vi "LS370Monitor_test.vi"(6 "still automatic":bool=TRUE, 8 "wait for T":bool=TRUE, 9 "Heater Off":bool=TRUE, 10 "Rate K/min":dbl, 11 "Setpoint LS370":dbl) -> (2 "Heater \nPower (W)":dbl, 3 "MC Temperature":dbl=291.191)   [LabVIEW 2016]
uses:
  Instrument_Setup_v2.vi
  data/Data_Display_global.vi
panel:
  out "MC Resistance":dbl=291.191
  out "FilmBurner heater (W)":dbl=1.0 format="%^_3e"
  in  "FilmBurner (mA)":dbl=1.0
  out "Nr. of cycles":i32
  in  "MC Thermometer":u16(ring)=2 items=["Speer S9905"=1, "Rox U02453"=2]
  out "Still heater (W)":dbl=1.0 format="%^_3e"
  in  "LS370 \nAuto Excitation":bool
  in  "Update every [ms]":dbl=1000.0 min=0.0 max=60000.0 step=500.0
  out "Auto\nExcitation":bool
  in  "Update every [ms] 2":dbl=60000.0 min=0.0 max=60000.0 step=500.0
  in  "Still value (mA)":dbl=3.0
  in  "T(K) still=on?":dbl=0.7
  out "?":bool
  out "?":bool
  out "?":bool
  in  "sweep\ntolerance %":dbl=0.1
  in  "stability \ntolerance (%)":dbl=0.5
  out "stability (K)":dbl
  out "Aktuelle Zeit":timestamp[](array[timestamp])
  out "Excitation AVS":dbl
  out "Excitation LS":dbl
  out "MC Temp kleiner als":dbl
  in  "stop":bool
  out "Temperature":cluster{timestamp[], dbl[]}[](graph)
  out "Heater Power":cluster{timestamp[], dbl[]}(graph)
  out "Offset new SP":dbl
  out "Heater Range":dbl
  out "P (Gain)":dbl
  out "I (Reset)":dbl
  out "D (Rate)":dbl
  out "HeaterTableLS370.txt":string caption="PID Table"
  out "Pfad zu HeaterTable":path=path "C:/01_Mischer_control/CryoTUM_Mischer_Version_2-0/HeaterTableLS370-highT"
  # "PID Control"
  # "Normal \noperation"
  # "Still control"
  # "0: Off\n1: 10mW\n2: 100mW\n3: 1.0W\n4: 10W"
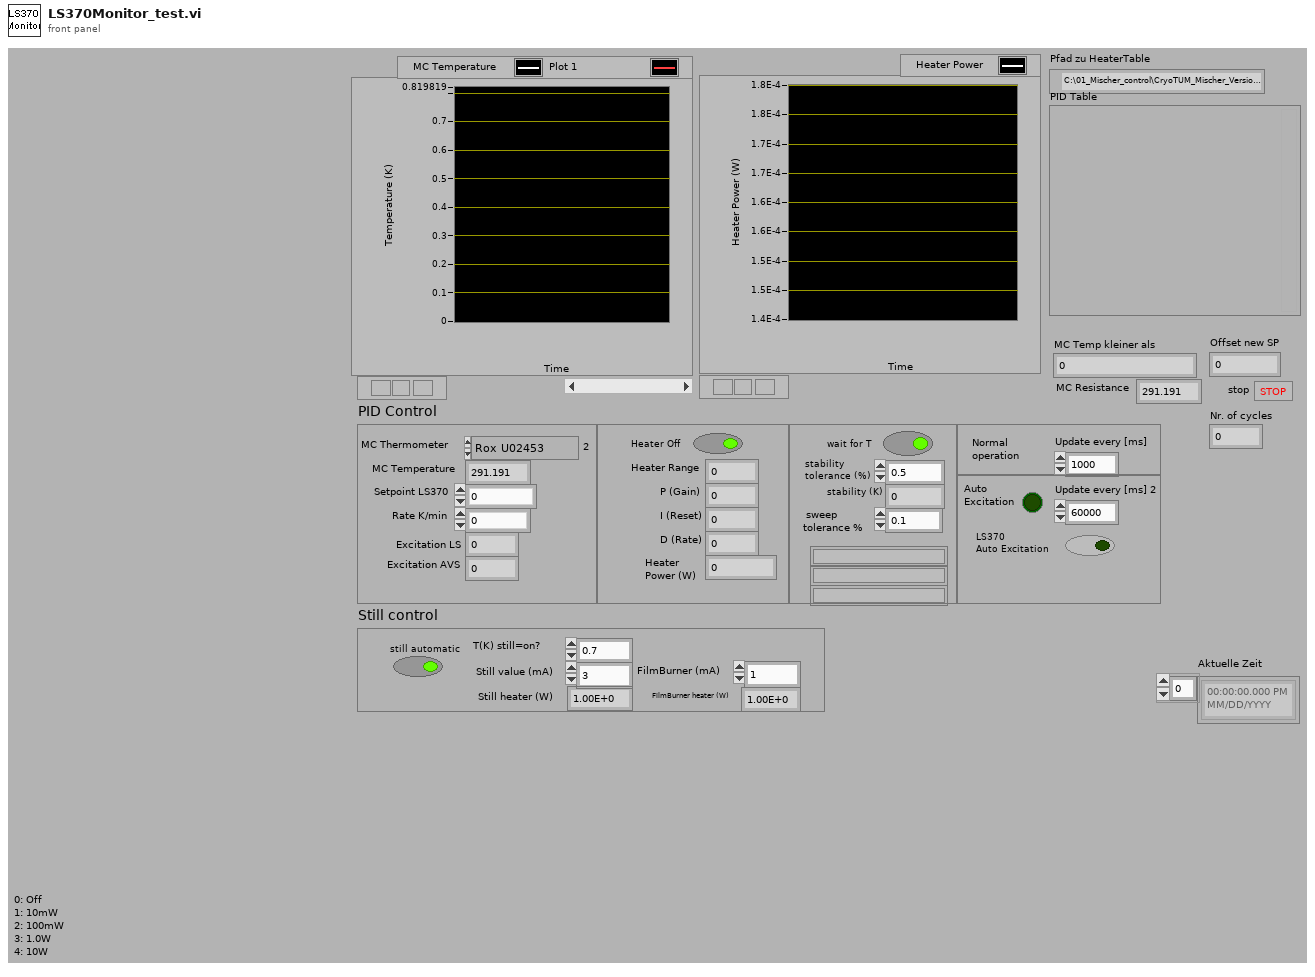
[diagram p1: front panel]
types:
  T1 = enum16{"open", "replace", "create", "open or create", "replace or create", "replace or create with confirmation"}
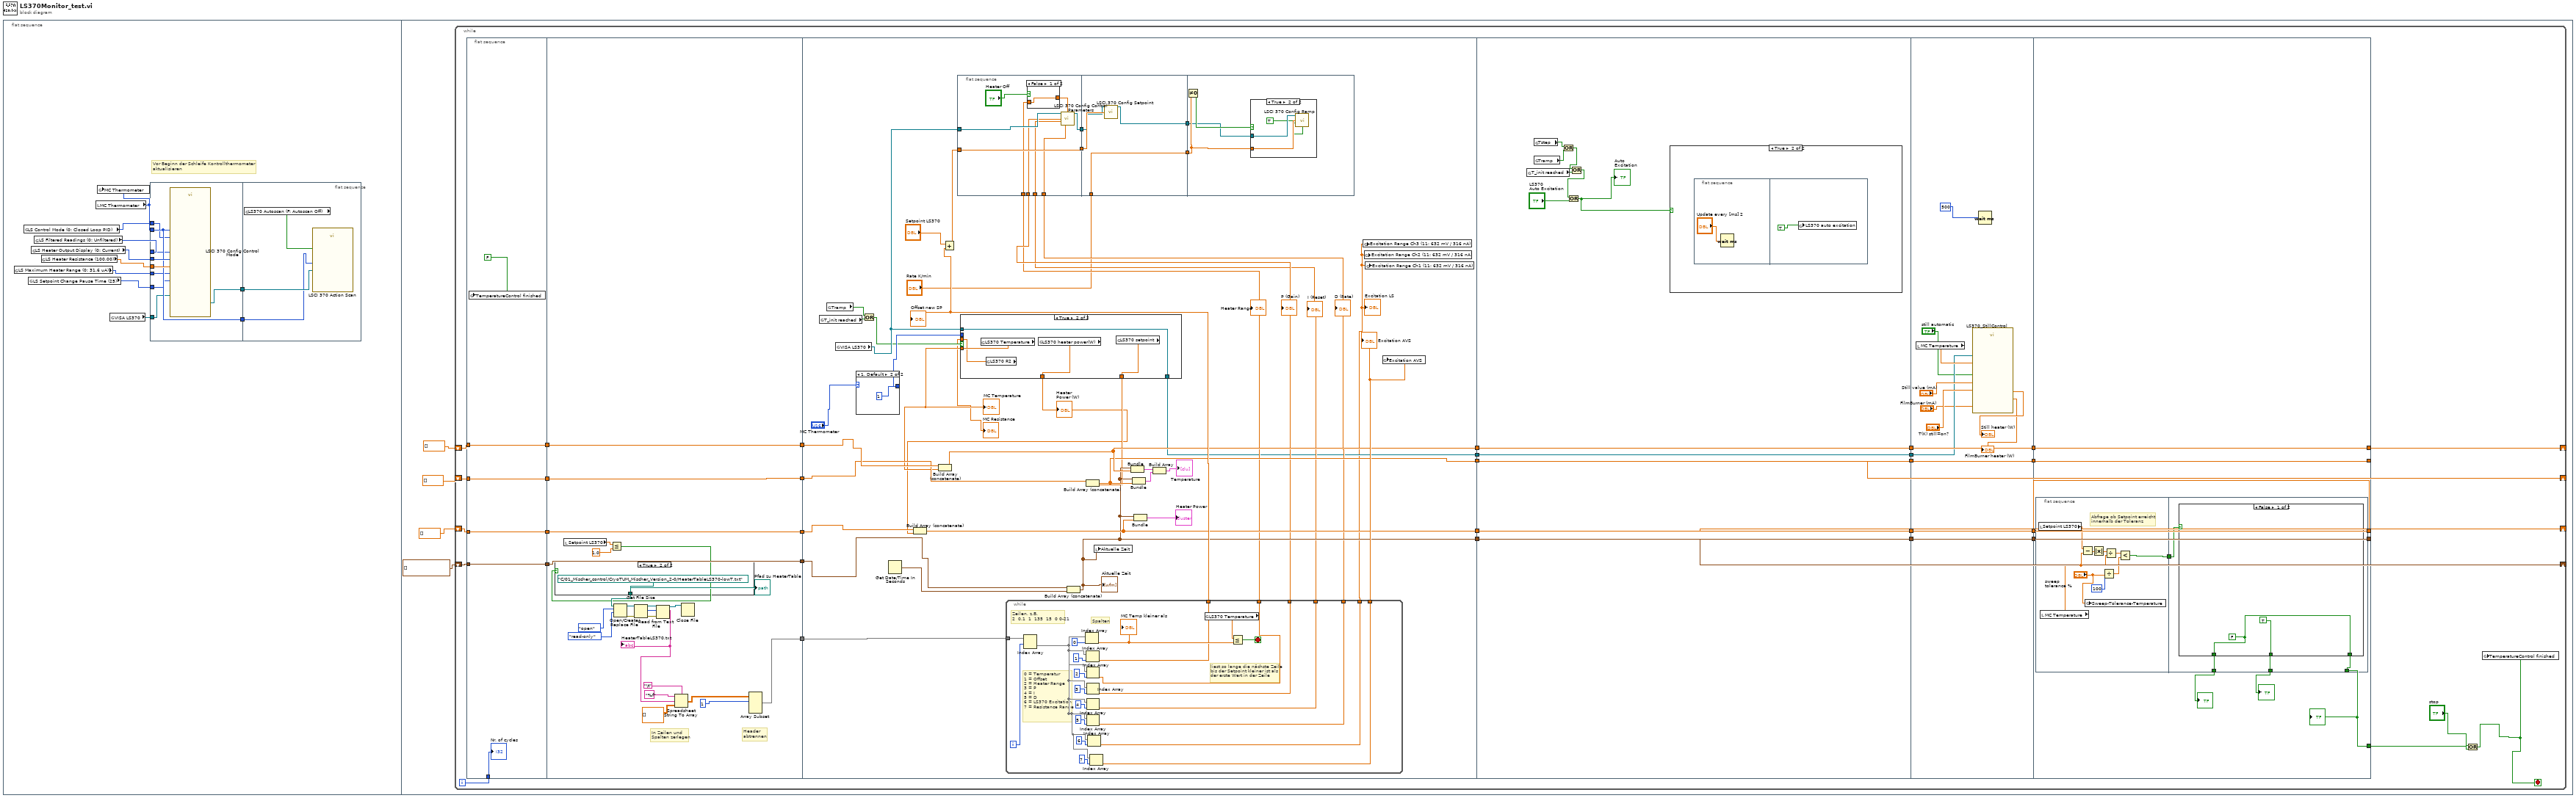
[diagram p0: block diagram]
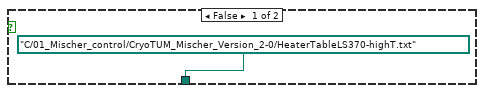
[diagram p2: hidden frame]
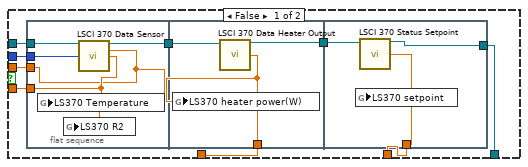
[diagram p3: hidden frame]
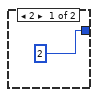
[diagram p4: hidden frame]
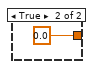
[diagram p5: hidden frame]
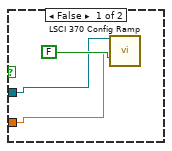
[diagram p6: hidden frame]
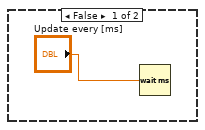
[diagram p7: hidden frame]
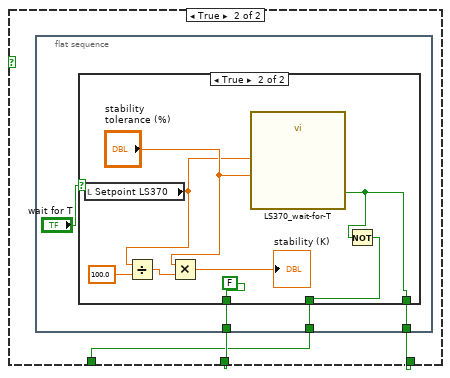
[diagram p8: hidden frame]
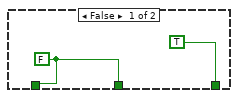
[diagram p9: hidden frame]
diagram:
  n1 = flat-sequence {
    frame #0 {
      # "Vor Beginn der Schleife Kontrollthermometer \naktualisieren"
      n2 = global read "Instrument_Setup_v2.vi" "LS Maximum Heater Range (0: 31.6 uA)"() -> (w2:u16)
      n3 = global read "Instrument_Setup_v2.vi" "LS Control Mode (0: Closed Loop PID)"() -> (w1:u16)
      n4 = global read "Instrument_Setup_v2.vi" "LS Setpoint Change Pause Time (25)"() -> (w3:i32)
      n5 = global read "Instrument_Setup_v2.vi" "LS Heater Output Display (0: Current)"() -> (w5:u16)
      n6 = global read "Instrument_Setup_v2.vi" "LS Filtered Readings (0: Unfiltered)"() -> (w6:u16)
      n7 = global read "Instrument_Setup_v2.vi" "LS Heater Resistance (100.00)"() -> (w4:dbl)
      n8 = local read "MC Thermometer"() -> (w7:u16)
      n9 = global write "Instrument_Setup_v2.vi" "MC Thermometer"(w7) -> ()
      n10 = global read "Instrument_Setup_v2.vi" "VISA LS370"() -> (w10:refnum<visa-resource-name>)
      n11 = flat-sequence {
        tunnel: w10 -> [w13]
        tunnel: w7 -> [w17]
        tunnel: w4 -> [w19]
        tunnel: w5 -> [w18]
        tunnel: [w17] -> w9
        tunnel: [w16] -> w8
        tunnel: w6 -> [w15]
        tunnel: w3 -> [w14]
        tunnel: w2 -> [w12]
        tunnel: w1 -> [w11]
        tunnel: w9 -> [w21]
        tunnel: w8 -> [w22]
        frame #0 {
          n12 = call "LSCI 370 Config Control Mode.vi"("VISA session"=w13, "Setpoint Change\nPause Time (25)"=w14, "Control Mode (0: Closed Loop PID)"=w11, "Channel (1)"=w17, "Filtered Readings (0: Unfiltered)"=w15, "Heater Output Display (0: Current)"=w18, "Heater Resistance (100.00)"=w19, "Maximum Heater Range (0: 31.6 uA)"=w12) -> ("dup VISA session"=w16:refnum<visa-resource-name>)  [unwired: 6 in, 1 out]
        }
        frame #1 {
          n13 = global read "Instrument_Setup_v2.vi" "LS370 Autoscan (F: Autoscan Off)"() -> (w20:bool)
          n14 = call "LSCI 370 Action Scan.vi"("VISA session"=w22, "Scan Channel (1)"=w21, "Autoscan (F: Autoscan Off)"=w20) -> ()  [unwired: 11 in, 2 out]
        }
      }
    }
    frame #1 {
      n15 = while {
        shift-right: [w54] -> _
        shift-left: dbl[] [] -> [w50]
        shift-right: [w53] -> _
        shift-left: timestamp[] [] -> [w49]
        shift-right: [w55] -> _
        shift-left: dbl[] [] -> [w51]
        shift-right: [w56] -> _
        shift-left: dbl[] [] -> [w52]
        i -> [w31]
        stop <- w29 stop-if-true
        n16 = flat-sequence {
          tunnel: w49 -> [w64]
          tunnel: w50 -> [w65]
          tunnel: w51 -> [w66]
          tunnel: w52 -> [w67]
          tunnel: [w67] -> w48
          tunnel: [w66] -> w47
          tunnel: [w65] -> w46
          tunnel: [w64] -> w45
          tunnel: w31 -> [w62]
          tunnel: [w76] -> w61
          tunnel: [w75] -> w60
          tunnel: [w74] -> w59
          tunnel: [w73] -> w58
          tunnel: [w72] -> w57
          tunnel: w48 -> [w75]
          tunnel: w47 -> [w74]
          tunnel: w46 -> [w73]
          tunnel: w45 -> [w72]
          tunnel: w61 -> [w131]
          tunnel: w60 -> [w122]
          tunnel: w59 -> [w121]
          tunnel: w58 -> [w120]
          tunnel: w57 -> [w119]
          tunnel: [w118] -> w40
          tunnel: [w117] -> w38
          tunnel: [w116] -> w36
          tunnel: [w115] -> w34
          tunnel: [w100] -> w32
          tunnel: w40 -> [w215]
          tunnel: [w215] -> w39
          tunnel: w38 -> [w214]
          tunnel: [w214] -> w37
          tunnel: w36 -> [w213]
          tunnel: [w213] -> w35
          tunnel: w34 -> [w212]
          tunnel: [w212] -> w33
          tunnel: w32 -> [w207]
          tunnel: [w207] -> w27
          tunnel: w39 -> [w231]
          tunnel: [w231] -> w44
          tunnel: w37 -> [w230]
          tunnel: [w230] -> w43
          tunnel: w35 -> [w229]
          tunnel: [w229] -> w42
          tunnel: w33 -> [w228]
          tunnel: [w228] -> w41
          tunnel: w27 -> [w224]
          tunnel: [w236] -> w53
          tunnel: [w237] -> w54
          tunnel: [w238] -> w55
          tunnel: [w239] -> w56
          tunnel: w44 -> [w239]
          tunnel: w43 -> [w238]
          tunnel: w42 -> [w237]
          tunnel: w41 -> [w236]
          tunnel: [w232] -> _
          tunnel: [w232] -> w30
          frame #0 {
            n17 = global write "Instrument_Setup_v2.vi" "TemperatureControl finished"(FALSE) -> ()
            "Nr. of cycles" <- w62
          }
          frame #1 {
            # "In Zeilen und \nSpalten zerlegen"
            # "Header\nabtrennen"
            n18 = local read "Setpoint LS370"() -> (w70:dbl)
            n19 = Less Or Equal?(x=w70, y=1.0) -> (x <= y?=w68:bool)
            n20 = case shown="True" w68 {
              tunnel: [path "C:/01_Mischer_control/CryoTUM_Mischer_Version_2-0/HeaterTableLS370-highT.txt" path "C:/01_Mischer_control/CryoTUM_Mischer_Version_2-0/HeaterTableLS370-lowT.txt"] -> w71
              frame False {
              }
              frame True {
              }
            }
            "Pfad zu HeaterTable" <- w71
            n21 = Open/Create/Replace File(file path (use dialog)=w71, operation (0:open)=T1."open", access (0:read/write)=enum16{"read/write", "read-only", "write-only"}."read-only") -> (refnum out=w86:refnum<file>, error out=w88:errorcluster)  [unwired: 3 in, 1 out]
            n22 = Get File Size(file=w86, error in=w88) -> (refnum out=w85:refnum<file>, size (in bytes)=w81:i64, 0:w87:errorcluster)
            n23 = Read from Text File(file (use dialog)=w85, count=w81, error in=w87) -> (refnum out=w84:refnum<file>, text=w80:string)  [unwired: 1 in, 2 out]
            "HeaterTableLS370.txt" <- w80
            n24 = Spreadsheet String To Array(delimiter (Tab)="\t", format string="%f", spreadsheet string=w80, array type (2D Dbl)=dbl[][] []) -> (array=w79:dbl[][])
            n25 = Close File(refnum=w84) -> ()  [unwired: 1 in, 2 out]
            n26 = Array Subset(array=w79, index (row)=1) -> (w76:dbl[][])  [unwired: 3 in]
          }
          frame #2 {
            n27 = global read "Data_Display_global.vi" "T_init reached"() -> (w97:bool)
            n28 = global read "Data_Display_global.vi" "Tramp"() -> (w96:bool)
            n29 = global read "Instrument_Setup_v2.vi" "VISA LS370"() -> (w102:refnum<visa-resource-name>)
            n30 = case shown="1, Default" "MC Thermometer" {
              tunnel: [2 1] -> w103
              frame 2 {
              }
              frame 1, Default {
              }
            }
            n31 = Or(x=w96, y=w97) -> (x .or. y?=w95:bool)
            n32 = Get Date/Time In Seconds() -> (seconds since 1Jan1904=w126:timestamp)
            n33 = flat-sequence {
              tunnel: [w167] -> w108
              tunnel: w113 -> [w165]
              tunnel: w112 -> [w164]
              tunnel: w111 -> [w163]
              tunnel: w110 -> [w162]
              tunnel: [w160] -> w107
              tunnel: w128 -> [w167]
              tunnel: w102 -> [w166]
              tunnel: w108 -> [w173]
              tunnel: [w170] -> w109
              tunnel: w107 -> [w172]
              tunnel: [w171] -> w106
              tunnel: "Rate K/min" -> [w170]
              tunnel: w109 -> [w175]
              tunnel: w106 -> [w174]
              frame #0 {
                n34 = case shown="False" "Heater Off" {
                  tunnel: w162 -> [w168 _]
                  tunnel: [w168 0.0] -> w161
                  frame False {
                  }
                  frame True {
                  }
                }
                n35 = call "LSCI 370 Config Control Parameters.vi"("VISA session"=w166, "Heater Range (0: Off)"=w161, "Gain (P) (10.000)"=w165, "Reset (I) (20)"=w164, "Rate (D) (0)"=w163) -> ("dup VISA session"=w160:refnum<visa-resource-name>)  [unwired: 9 in, 1 out]
              }
              frame #1 {
                n36 = call "LSCI 370 Config Setpoint.vi"("VISA session"=w172, "Setpoint (0.00000E+0)"=w173) -> ("dup VISA session"=w171:refnum<visa-resource-name>)  [unwired: 12 in, 1 out]
              }
              frame #2 {
                n37 = Not Equal To 0?(x=w175) -> (x != 0?=w176:bool)
                n38 = case shown="True" w176 {
                  tunnel: w174 -> [w178 w182]
                  tunnel: w175 -> [w177 w181]
                  frame False {
                    n39 = call "LSCI 370 Config Ramp.vi"("VISA session"=w178, "Rate Value (0.001)"=w177, "Ramping On/Off (F: Ramping Off)"=FALSE) -> ()  [unwired: 11 in, 2 out]
                  }
                  frame True {
                    n40 = call "LSCI 370 Config Ramp.vi"("VISA session"=w182, "Rate Value (0.001)"=w181, "Ramping On/Off (F: Ramping Off)"=TRUE) -> ()  [unwired: 11 in, 2 out]
                  }
                }
              }
            }
            n41 = case shown="True" w95 {
              tunnel: w103 -> [w138 _]
              tunnel: w102 -> [w137 w153]
              tunnel: [w136 w154] -> w101
              tunnel: [w135 w153] -> w100
              tunnel: [w134 w156] -> w99
              tunnel: [w133 w155] -> w98
              tunnel: [w132 w152] -> w94
              frame False {
                n42 = flat-sequence {
                  tunnel: w138 -> [w145]
                  tunnel: w137 -> [w144]
                  tunnel: [w143] -> w140
                  tunnel: [w142] -> w134
                  tunnel: [w141] -> w132
                  tunnel: w140 -> [w148]
                  tunnel: [w146] -> w133
                  tunnel: [w147] -> w139
                  tunnel: [w149] -> w136
                  tunnel: w139 -> [w151]
                  tunnel: [w150] -> w135
                  frame #0 {
                    n43 = call "LSCI 370 Data Sensor.vi"("VISA session"=w144, "Channel (1)"=w145) -> ("dup VISA session"=w143:refnum<visa-resource-name>, "Resistance Reading"=w141:dbl, "Kelvin Reading"=w142:dbl)  [unwired: 9 in, 2 out]
                    n44 = global write "Data_Display_global.vi" "LS370 Temperature"(w142) -> ()
                    n45 = global write "Data_Display_global.vi" "LS370 R2"(w141) -> ()
                  }
                  frame #1 {
                    n46 = call "LSCI 370 Data Heater Output.vi"("VISA session"=w148) -> ("dup VISA session"=w147:refnum<visa-resource-name>, "Heater Output"=w146:dbl)  [unwired: 12 in, 1 out]
                    n47 = global write "Data_Display_global.vi" "LS370 heater power(W)"(w146) -> ()
                  }
                  frame #2 {
                    n48 = call "LSCI 370 Status Setpoint.vi"("VISA session"=w151) -> ("dup VISA session"=w150:refnum<visa-resource-name>, "Setpoint (0.00000E+0)"=w149:dbl)  [unwired: 12 in, 1 out]
                    n49 = global write "Data_Display_global.vi" "LS370 setpoint"(w149) -> ()
                  }
                }
              }
              frame True {
                n50 = global read "Data_Display_global.vi" "LS370 Temperature"() -> (w156:dbl)
                n51 = global read "Data_Display_global.vi" "LS370 R2"() -> (w152:dbl)
                n52 = global read "Data_Display_global.vi" "LS370 heater power(W)"() -> (w155:dbl)
                n53 = global read "Data_Display_global.vi" "LS370 setpoint"() -> (w154:dbl)
              }
            }
            "MC Temperature" <- w99
            "Heater \nPower (W)" <- w98
            "MC Resistance" <- w94
            n54 = Build Array (concatenate)(w120, w98) -> (w116:dbl[])
            n55 = Build Array (concatenate)(w122, w99) -> (w118:dbl[])
            n56 = while {
              tunnel: w131 -> [w203]
              tunnel: [w194] -> w129
              tunnel: [w192] -> w110
              tunnel: [w191] -> w113
              tunnel: [w190] -> w112
              tunnel: [w189] -> w111
              tunnel: [w187] -> w93
              tunnel: [w184] -> w127
              i -> [w202]
              stop <- w196 stop-if-true
              # "0 = Temperatur\n1 = Offset\n2 = Heater Range\n3 = P\n4 = I\n5 = D\n6 = LS370 Excitation\n7 = Resistance Range"
              # "liest so lange die nächste Zeile\nbis der Setpoint kleiner ist als \nder erste Wert in der Zeile"
              # "Zeilen, z.B. \n2  0.1  1  135  15  0 0-21"
              # "Spalten"
              n57 = Index Array(array=w203, index (row)=w202) -> (element=w185:dbl[])  [unwired: 1 in]
              n58 = Index Array(array=w185, index=0) -> (element=w195:dbl)
              "MC Temp kleiner als" <- w195
              n59 = Index Array(array=w185, index=1) -> (element=w194:dbl)
              n60 = Index Array(array=w185, index=2) -> (element=w192:dbl)
              n61 = Index Array(array=w185, index=3) -> (element=w191:dbl)
              n62 = Index Array(array=w185, index=4) -> (element=w190:dbl)
              n63 = Index Array(array=w185, index=5) -> (element=w189:dbl)
              n64 = Index Array(array=w185, index=6) -> (element=w187:dbl)
              n65 = Index Array(array=w185, index=7) -> (element=w184:dbl)
              n66 = global read "Data_Display_global.vi" "LS370 Temperature"() -> (w183:dbl)
              n67 = Less Or Equal?(x=w183, y=w195) -> (x <= y?=w196:bool)
            }
            "Offset new SP" <- w129
            "Heater Range" <- w110
            "P (Gain)" <- w113
            "I (Reset)" <- w112
            "D (Rate)" <- w111
            "Excitation LS" <- w93
            "Excitation AVS" <- w127
            n68 = Add(x="Setpoint LS370", y=w129) -> (x+y=w128:dbl)
            n69 = Build Array (concatenate)(w119, w126) -> (w115:timestamp[])
            "Aktuelle Zeit" <- w115
            n70 = Build Array (concatenate)(w121, w101) -> (w117:dbl[])
            n71 = local write "Aktuelle Zeit"(w115) -> ()
            n72 = Bundle(w115, w118) -> (w125:cluster{timestamp[], dbl[]})  [unwired: 1 in]
            n73 = Bundle(w115, w117) -> (w123:cluster{timestamp[], dbl[]})  [unwired: 1 in]
            n74 = Bundle(w115, w116) -> (→"Heater Power":cluster{timestamp[], dbl[]})  [unwired: 1 in]
            n75 = Build Array(w125, w123) -> (→"Temperature":cluster{timestamp[], dbl[]}[])
            n76 = global write "Instrument_Setup_v2.vi" "Excitation Range Ch3 (11: 632 mV / 316 nA)"(w93) -> ()
            n77 = global write "Instrument_Setup_v2.vi" "Excitation Range Ch2 (11: 632 mV / 316 nA)"(w93) -> ()
            n78 = global write "Instrument_Setup_v2.vi" "Excitation Range Ch1 (11: 632 mV / 316 nA)"(w93) -> ()
            n79 = global write "Instrument_Setup_v2.vi" "Excitation AVS"(w127) -> ()
          }
          frame #3 {
            n80 = global read "Data_Display_global.vi" "T_init reached"() -> (w211:bool)
            n81 = global read "Data_Display_global.vi" "Tstep"() -> (w206:bool)
            n82 = global read "Data_Display_global.vi" "Tramp"() -> (w205:bool)
            n83 = Or(x=w206, y=w205) -> (x .or. y?=w204:bool)
            n84 = Or(x=w204, y=w211) -> (x .or. y?=w209:bool)
            n85 = Or(x=w209, y="LS370 \nAuto Excitation") -> (x .or. y?=w208:bool)
            "Auto\nExcitation" <- w208
            n86 = case shown="True" w208 {
              frame False {
                n87 = Wait (ms)(milliseconds to wait="Update every [ms]") -> ()  [unwired: 1 out]
              }
              frame True {
                n88 = flat-sequence {
                  frame #0 {
                    n89 = Wait (ms)(milliseconds to wait="Update every [ms] 2") -> ()  [unwired: 1 out]
                  }
                  frame #1 {
                    n90 = global write "Data_Display_global.vi" "LS370 auto excitation"(TRUE) -> ()
                  }
                }
              }
            }
          }
          frame #4 {
            n91 = local read "MC Temperature"() -> (w225:dbl)
            n92 = call "LS370_StillControl.vi"("LS370 ch2 K"=w225, "FilmBurner value (mA)"="FilmBurner (mA)", "T(K) still=on?"="T(K) still=on?", "Still value (mA)"="Still value (mA)", "still automatic"="still automatic", "GPIB"=w224) -> ("FilmBurner (W)"=→"FilmBurner heater (W)":dbl, "Still heater (W)"=→"Still heater (W)":dbl)  [unwired: 4 in]
            n93 = Wait (ms)(milliseconds to wait=500) -> ()  [unwired: 1 out]
          }
          frame #5 {
            n94 = flat-sequence {
              tunnel: [w241] -> w235
              tunnel: [w252] -> w232
              tunnel: w235 -> [w251]
              tunnel: [w250] -> w234
              tunnel: [w249] -> w233
              frame #0 {
                # "Abfrage ob Setpoint erreicht\ninnerhalb der Toleranz"
                n95 = local read "Setpoint LS370"() -> (w243:dbl)
                n96 = local read "MC Temperature"() -> (w242:dbl)
                n97 = Subtract(x=w243, y=w242) -> (x-y=w245:dbl)
                n98 = global write "Instrument_Setup_v2.vi" "Sweep-Tolerance-Temperature"("sweep\ntolerance %") -> ()
                n99 = Absolute Value(x=w245) -> (abs(x)=w246:dbl)
                n100 = Divide(x="sweep\ntolerance %", y=100) -> (x/y=w248:dbl)
                n101 = Divide(x=w246, y=w242) -> (x/y=w247:dbl)
                n102 = Less?(x=w247, y=w248) -> (x < y?=w241:bool)
              }
              frame #1 {
                n103 = case shown="False" w251 {
                  tunnel: [w253 w257] -> w252
                  tunnel: [TRUE w256] -> w250
                  tunnel: [w253 w255] -> w249
                  frame False {
                    w253 = FALSE
                  }
                  frame True {
                    n104 = flat-sequence {
                      tunnel: [w260] -> w257
                      tunnel: [w259] -> w256
                      tunnel: [w258] -> w255
                      frame #0 {
                        n105 = case shown="True" "wait for T" {
                          tunnel: [TRUE ("T innerhalb Toleranz") w265] -> w260
                          tunnel: [w262 FALSE] -> w259
                          tunnel: [w262 w264] -> w258
                          frame False {
                            w262 = FALSE
                          }
                          frame True {
                            n106 = local read "Setpoint LS370"() -> (w267:dbl)
                            n107 = Divide(x=w267, y=100.0) -> (x/y=w269:dbl)
                            n108 = Multiply(x="stability \ntolerance (%)", y=w269) -> (x*y=→"stability (K)":dbl)
                            n109 = call "LS370_wait-for-T.vi"("Toleranz (%)"="stability \ntolerance (%)", "T_target"=w267) -> ("T innerhalb Toleranz"=w265:bool)  [unwired: 9 in]
                            n110 = Not(x=w265) -> (.not. x?=w264:bool)
                          }
                        }
                      }
                    }
                  }
                }
              }
            }
            "?" <- w232
            "?" <- w234
            "?" <- w233
          }
        }
        n111 = Or(x="stop", y=w30) -> (x .or. y?=w29:bool)
        n112 = global write "Instrument_Setup_v2.vi" "TemperatureControl finished"(w29) -> ()
      }
    }
  }
